vi "SetupStriptest.vi"(3 "Probe Card Channels":i32=1) -> (1 "Continue?":bool)   [LabVIEW 2018]
uses:
  ProbePlan/ProbePlanParams.vi
  general_VIs/globals/QC_RunInformation.vi
  general_VIs/globals/QC_MeasurementSetup.vi
panel:
  in  "Sensor Bias":dbl=-150.0
  out "Instructions:":string="- configure Arduino edgesense; optional testing of edgesense                                        - define probing range\n- select LCR meter, bias, and IV supply; configure if necessary                                         - adjust measurement parameters\n- select operator                                                                                                          - select tests included"
  in  "Bias Supply":u16(ring) items=["Dont set here"]
  in  "Test Button":bool
  in  "Resistance Y/N":bool=TRUE
  in  "Capacitance Y/N":bool=TRUE
  in  "Pinholes Y/N":bool=TRUE
  in  "High Step":i32=1000
  in  "Base Step":i32=1000
  in  "High Ramp":dbl=100.0
  in  "Base Ramp":dbl=10.0
  in  "High V":dbl=100.0
  in  "Base V":dbl=10.0
  in  "Quit":bool
  in  "Continue":bool
  in  "Settings Button":bool
  in  "T/RH Readout":enum16{"Arduino Uno", "Nothing"}(ring)=enum."Nothing"
  in  "LCR meter:":u16(ring) items=["Dont set here"]
  in  "IV Supply:":u16(ring) items=["Dont set here"]
  in  "Operator:":u32(ring) items=["Jiri Kv", "Saevar", "Maurice", "Rick", "Dave", "Bart", "Miguel", "Christoph", "Other..."]
  out "DataBase Serial No.:":string="DatabaseSerialNo"
  out "Manufacturer:":string="Hamamatsu"
  out "Device Category:":string
  out "Manufacturer Serial No.:":string="ManufactSerialNo"
  out "Region4":string
  out "Region3":string
  out "Region2":string
  out "Region":string
  in  "From4":u16(ring)
  in  "From3":u16(ring)
  in  "From2":u16(ring)
  in  "From":u16(ring)
  in  "To4":u16(ring)
  in  "To3":u16(ring)
  in  "To2":u16(ring)
  in  "To":u16(ring)
  in  "Enable4":bool
  in  "Enable3":bool
  in  "Enable2":bool
  in  "Enable1":bool
  # "Setup Striptest"
  # "Define Probe Range"
  # "Measurement Parameters"
  # "Volts"
  # "Base Voltage Settings"
  # "High Voltage Settings"
  # "Volts"
  # "Volts"
  # "Volts/step"
  # "Volts/step"
  # "millisec"
  # "millisec"
  # "DUT & Test Description"
  # "Tests Included"
  # "Hardware"
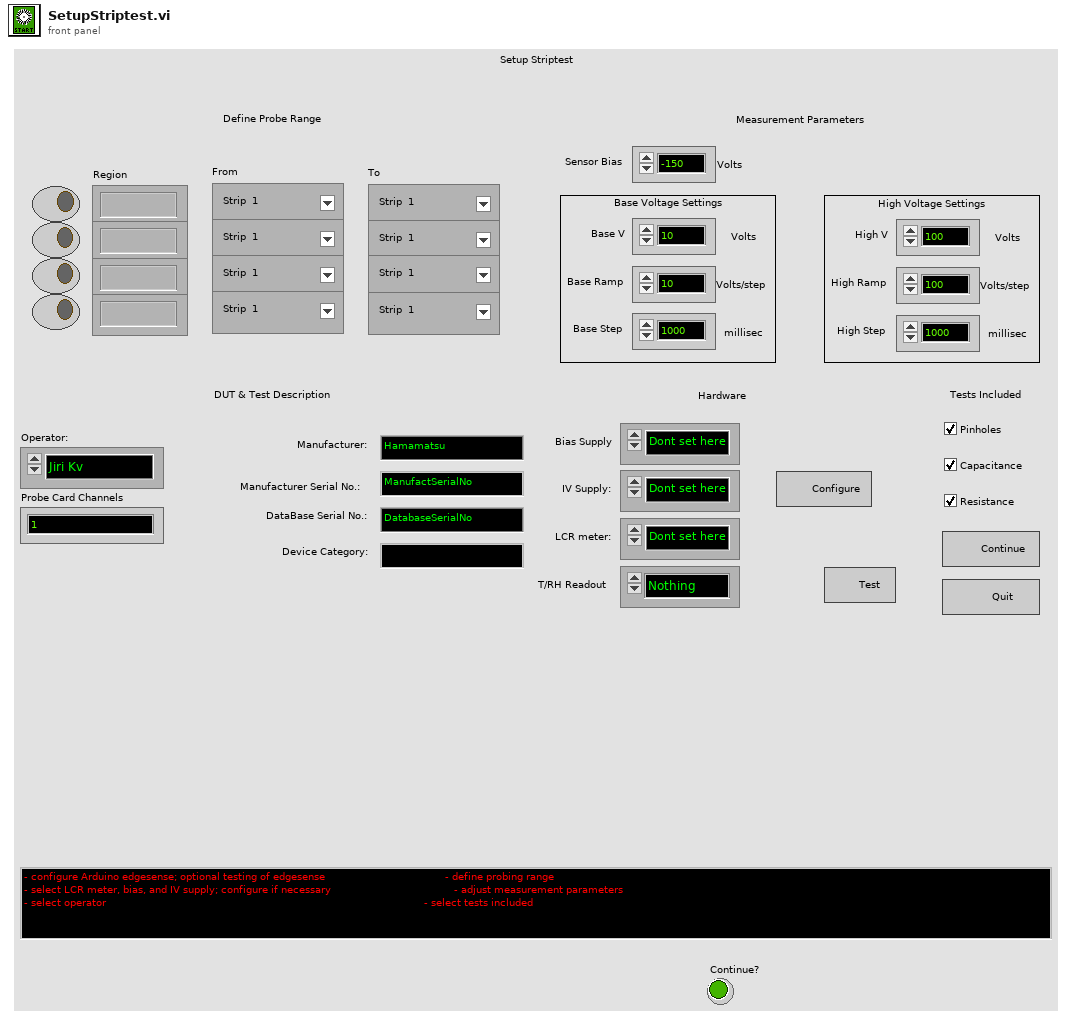
[diagram p1: front panel]
types:
  T1 = cluster{"Strip Number OUT":i32, "X0":i32, "Y0":i32, "X1":i32, "Y1":i32, "Xref":dbl, "Yref":dbl, "ProbePlan type":u32, "Inner pads offset":ext, "Outer pads offset":ext, "l_inner":ext, "l_outer":ext, "strip numbering":u16, "Device Orientation":ext, "Stagger offset":i32, "Yoffset":dbl, "Strip pitch":dbl, "Fiducail separation":dbl, "Radius":ext, "Relative strip angles":dbl, "Probeplan description":string, "ProbePlan array":cluster{"Region":string, "ProbePoints":cluster{"X":dbl, "Y":dbl, "Label":string, "CardViable?":bool}[]}[], "Test ProbePoints":cluster{"Regions Enabled":bool[], "From index":u32[], "To index":u32[]}}
  T2 = cluster{"Region":string, "ProbePoints":cluster{"X":dbl, "Y":dbl, "Label":string, "CardViable?":bool}[]}[]
  T3 = cluster{"Sensor Serial No.:":string, "Wafer Serial No.:":string, "Batch:":string, "Manufacturer:":string, "Device Category:":string, "Database Serial No.:":string, "Initiated:":string, "Test":string, "Instruments used:":string, "Probeplan used:":string, "End of Run comment:":string, "User:":string}
  T4 = cluster{"Bias Supply":refnum<class "SupplyControl.lvclass">, "SMU":refnum<class "SupplyControl.lvclass">, "LCR":refnum<class "LCRControl.lvclass">, "Probe Card Channels":i32, "Bias Voltage [V]":dbl, "First strip":i32, "Last strip":i32, "Base Voltage [V]":dbl, "Base Ramp Step [V]":dbl, "Base Ramp Interval [ms]":u32, "High Voltage [V]":dbl, "High Ramp Step [V]":dbl, "High Ramp Interval [ms]":u32, "Single Needle":bool, "Temperature Readout":enum16{"Read Arduino", "Enter manually"}, "Arduino":refnum<class "ArduinoControl.lvclass">, "Fraction of good strips [%]":dbl, "ProbeStation":refnum<class "ProbeStationControl.lvclass">, "AC frequency [Hz]":i32, "Switching":refnum<class "Switching.lvclass">, "Matrix used?":bool, "Matrix X Channels":cluster{"Bias Supply / SMU LO":i32, "Bias Supply / SMU HI":i32, "CV Box LO":i32, "CV Box HI":i32, "CV Box LO IN":i32, "CV Box HI IN":i32, "Volt meter LO":i32, "Volt meter HI":i32, "Mux1 C1":i32, "Mux1 C2":i32, "Mux2 C1":i32, "Mux2 C2":i32}, "Pinholes Y/N":bool, "Capacitance Y/N":bool, "Resistance Y/N":bool}
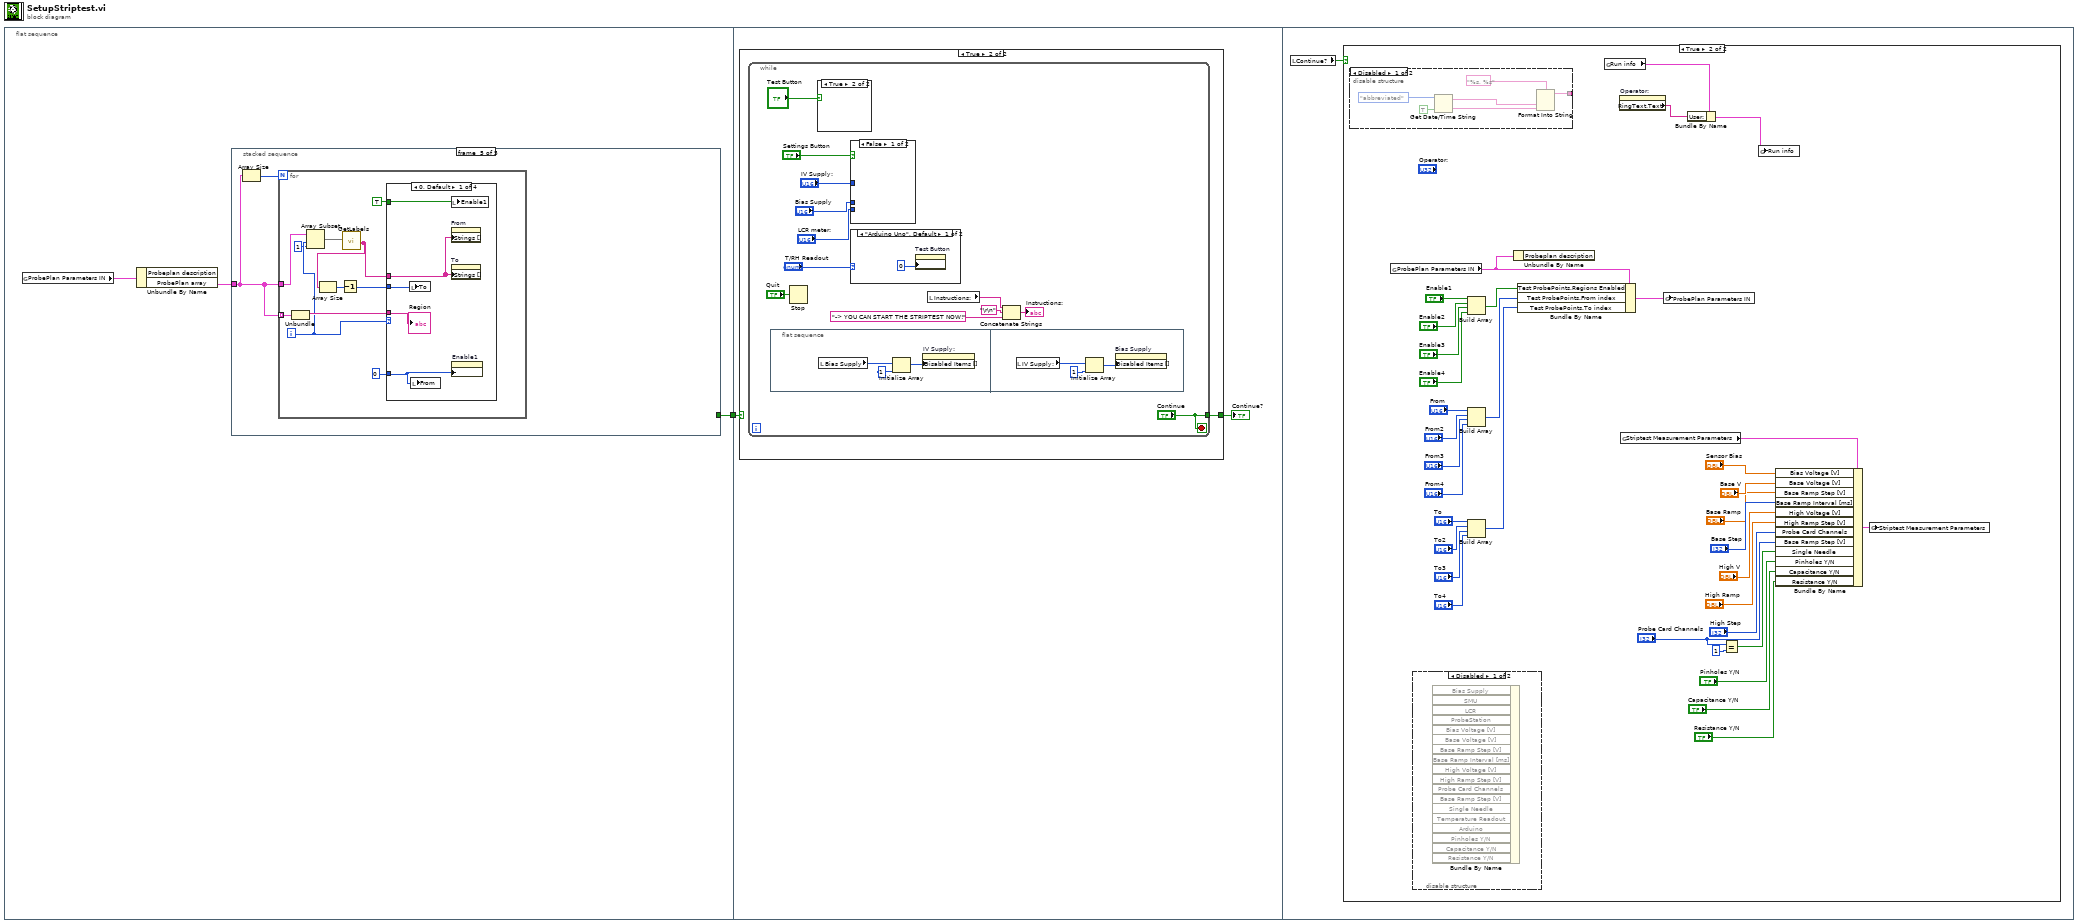
[diagram p0: block diagram]
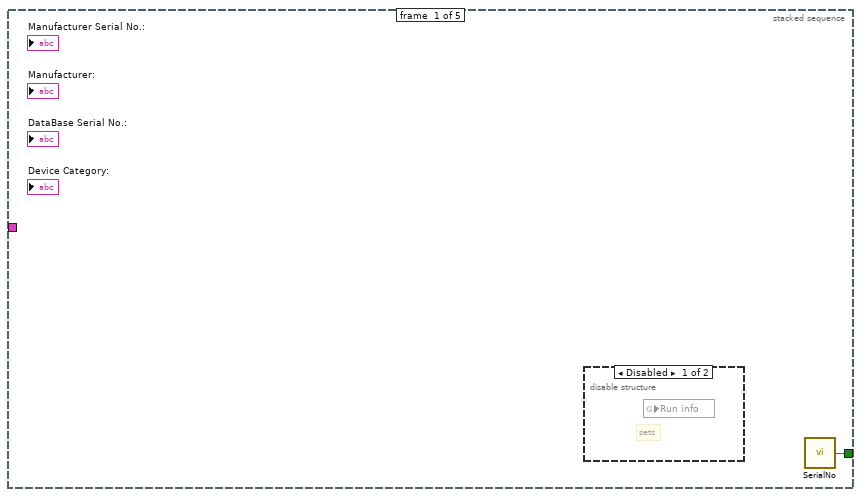
[diagram p2: hidden frame]
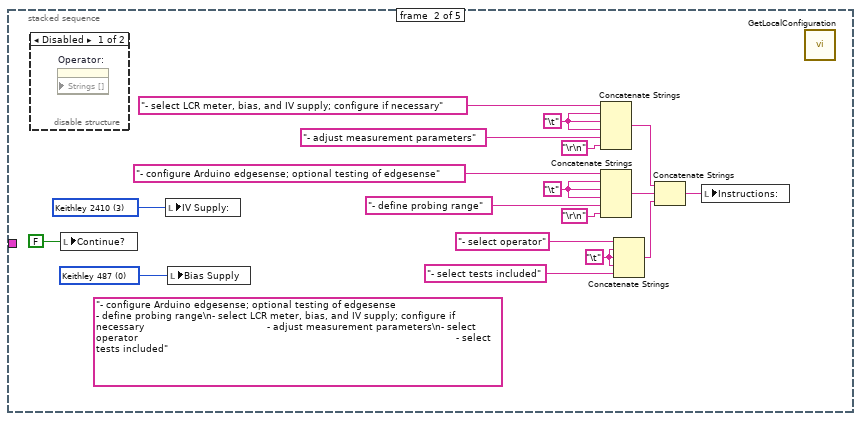
[diagram p4: hidden frame]
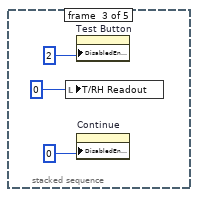
[diagram p6: hidden frame]
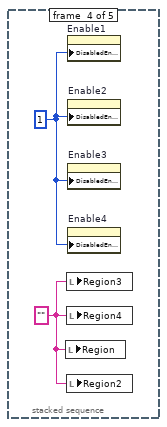
[diagram p7: hidden frame]
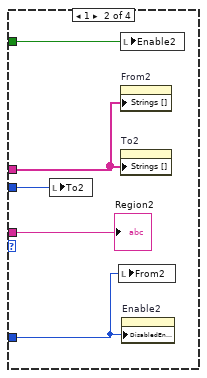
[diagram p8: hidden frame]
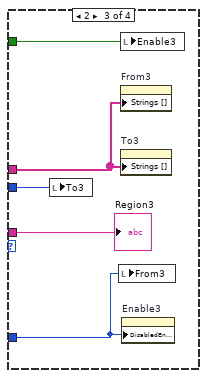
[diagram p9: hidden frame]
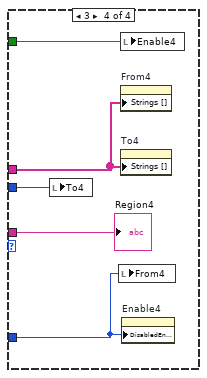
[diagram p10: hidden frame]
diagram:
  n1 = flat-sequence {
    tunnel: [w2] -> w1
    tunnel: w1 -> [w62]
    frame #0 {
      n2 = global read "ProbePlanParams.vi" "ProbePlan Parameters IN"() -> (w4:T1)
      n3 = Unbundle By Name(w4) -> ("ProbePlan array"=w3:T2)  [unwired: 1 out]
      n4 = stacked-sequence {
        tunnel: w3 -> [_ _ _ _ w29]
        tunnel: [w5 _ _ _ _] -> w2
        frame #0 {
          n5 = disable-structure shown="Disabled" {
            frame Disabled {
              # "sets"
              n6 = global read "QC_RunInformation.vi" "Run info"() -> ()  [unwired: 1 in]
            }
            frame Enabled {
            }
          }
          n7 = call "SerialNo.vi"() -> ("Continue?"=w5:bool)  [unwired: 5 in]
        }
        frame #1 {
          w14 = "\t"
          w16 = "\t"
          w20 = "\t"
          (unwired) "- configure Arduino edgesense; optional testing of edgesense                                        - define probing range\n- select LCR meter, bias, and IV supply; configure if necessary                                         - adjust measurement parameters\n- select operator                                                                                                          - select tests included" ("Instructions:")
          w21 = u16 0 items=["Keithley 487", "Keithley 6517", "Keithley 236/237", "Keithley 2410"] ("Supply:")
          w22 = u16 3 items=["Keithley 487", "Keithley 6517", "Keithley 236/237", "Keithley 2410"] ("Supply:")
          n8 = disable-structure shown="Disabled" {
            frame Disabled {
              n9 = property on="Operator:" class="Ring (strict)" props=["Strings []"]() -> ()  [unwired: 3 in, 2 out]
            }
            frame Enabled {
            }
          }
          n10 = local write "Continue?"(FALSE ("Continue?")) -> ()
          n11 = local write "IV Supply:"(w22) -> ()
          n12 = local write "Bias Supply"(w21) -> ()
          n13 = Concatenate Strings("- select LCR meter, bias, and IV supply; configure if necessary", w16, w16, w16, "- adjust measurement parameters", "\r\n") -> (w9:string)
          n14 = Concatenate Strings("- configure Arduino edgesense; optional testing of edgesense", w20, w20, w20, "- define probing range", "\r\n") -> (w10:string)
          n15 = Concatenate Strings("- select operator", w14, w14, w14, "- select tests included") -> (w11:string)
          n16 = Concatenate Strings(w9, w10, w11) -> (w8:string)
          n17 = local write "Instructions:"(w8) -> ()
          n18 = call "GetLocalConfiguration.vi"() -> ()  [unwired: 3 in, 1 out]
        }
        frame #2 {
          n19 = local write "T/RH Readout"(0) -> ()
          n20 = property on="Test Button" class="Bool"("DisabledEnum"=2) -> ()  [unwired: 2 in, 2 out]
          n21 = property on="Continue" class="Bool"("DisabledEnum"=u8 0 ("Disabled")) -> ()  [unwired: 2 in, 2 out]
        }
        frame #3 {
          w28 = "" ("Region")
          w27 = u8 1 ("Disabled")
          n22 = local write "Region"(w28) -> ()
          n23 = local write "Region3"(w28) -> ()
          n24 = local write "Region4"(w28) -> ()
          n25 = local write "Region2"(w28) -> ()
          n26 = property on="Enable1" class="Bool (strict)"("DisabledEnum"=w27) -> ()  [unwired: 2 in, 2 out]
          n27 = property on="Enable2" class="Bool (strict)"("DisabledEnum"=w27) -> ()  [unwired: 2 in, 2 out]
          n28 = property on="Enable3" class="Bool (strict)"("DisabledEnum"=w27) -> ()  [unwired: 2 in, 2 out]
          n29 = property on="Enable4" class="Bool (strict)"("DisabledEnum"=w27) -> ()  [unwired: 2 in, 2 out]
        }
        frame #4 {
          n30 = Array Size(array=w29) -> (size(s)=w30:i32)
          n31 = for {
            N: w30 -> [_]
            tunnel: w29 -> [w34]
            tunnel: w29 -> [w39] mode=indexing
            i -> [w33]
            n32 = Unbundle(w39) -> ("Region"=w38:string)  [unwired: 1 out]
            n33 = Array Subset(array=w34, index=w33, length=1) -> (w31:T2)
            n34 = call "GetLabels.vi"("Array"=w31) -> ("Strip Labels"=w35:string[])  [unwired: 3 out]
            n35 = Array Size(array=w35) -> (size(s)=w37:i32)
            n36 = Decrement(x=w37) -> (x-1=w36:i32)
            n37 = case shown="0, Default" w33 {
              tunnel: TRUE -> [w46 w50 w56 w61]
              tunnel: 0 -> [w42 w47 w52 w57]
              tunnel: w38 -> [w44 w49 w54 w59]
              tunnel: w35 -> [w43 w48 w53 w58]
              tunnel: w36 -> [w45 w51 w55 w60]
              frame 0, Default {
                n38 = local write "To"(w45) -> ()
                n39 = local write "From"(w42) -> ()
                n40 = local write "Enable1"(w46) -> ()
                n41 = property on="From" class="Ring (strict)"("Strings []"=w43) -> ()  [unwired: 2 in, 2 out]
                n42 = property on="To" class="Ring (strict)"("Strings []"=w43) -> ()  [unwired: 2 in, 2 out]
                n43 = property on="Enable1" class="Bool (strict)"("DisabledEnum"=w42) -> ()  [unwired: 2 in, 2 out]
                "Region" <- w44
              }
              frame 1 {
                n44 = local write "To2"(w51) -> ()
                n45 = local write "From2"(w47) -> ()
                n46 = local write "Enable2"(w50) -> ()
                n47 = property on="From2" class="Ring (strict)"("Strings []"=w48) -> ()  [unwired: 2 in, 2 out]
                n48 = property on="To2" class="Ring (strict)"("Strings []"=w48) -> ()  [unwired: 2 in, 2 out]
                n49 = property on="Enable2" class="Bool (strict)"("DisabledEnum"=w47) -> ()  [unwired: 2 in, 2 out]
                "Region2" <- w49
              }
              frame 2 {
                n50 = local write "To3"(w55) -> ()
                n51 = local write "From3"(w52) -> ()
                n52 = local write "Enable3"(w56) -> ()
                n53 = property on="From3" class="Ring (strict)"("Strings []"=w53) -> ()  [unwired: 2 in, 2 out]
                n54 = property on="To3" class="Ring (strict)"("Strings []"=w53) -> ()  [unwired: 2 in, 2 out]
                n55 = property on="Enable3" class="Bool (strict)"("DisabledEnum"=w52) -> ()  [unwired: 2 in, 2 out]
                "Region3" <- w54
              }
              frame 3 {
                n56 = local write "To4"(w60) -> ()
                n57 = local write "From4"(w57) -> ()
                n58 = local write "Enable4"(w61) -> ()
                n59 = property on="From4" class="Ring (strict)"("Strings []"=w58) -> ()  [unwired: 2 in, 2 out]
                n60 = property on="To4" class="Ring (strict)"("Strings []"=w58) -> ()  [unwired: 2 in, 2 out]
                n61 = property on="Enable4" class="Bool (strict)"("DisabledEnum"=w57) -> ()  [unwired: 2 in, 2 out]
                "Region4" <- w59
              }
            }
          }
        }
      }
    }
    frame #1 {
      n62 = case shown="True" w62 {
        selector: w62 -> [w64 _]
        tunnel: [w64 w65] -> w63
        frame False {
        }
        frame True {
          n63 = while {
            tunnel: ["Continue"] -> w65
            stop <- "Continue" stop-if-true
            n64 = flat-sequence {
              frame #0 {
                n65 = local read "Bias Supply"() -> (w79:u16)
                n66 = Initialize Array(w79, 1) -> (w80:u16[])
                n67 = property on="IV Supply:" class="Ring (strict)"("Disabled Items []"=w80) -> ()  [unwired: 2 in, 2 out]
              }
              frame #1 {
                n68 = local read "IV Supply:"() -> (w84:u16)
                n69 = Initialize Array(w84, 1) -> (w82:u16[])
                n70 = property on="Bias Supply" class="Ring (strict)"("Disabled Items []"=w82) -> ()  [unwired: 2 in, 2 out]
              }
            }
            n71 = Stop(stop? (T)="Quit") -> ()
            n72 = case shown="True" "Test Button" {
              frame False {
              }
              frame True {
              }
            }
            n73 = case shown="False" "Settings Button" {
              tunnel: "IV Supply:" -> [_ _]
              tunnel: "LCR meter:" -> [_ _]
              tunnel: "Bias Supply" -> [_ _]
              frame False {
              }
              frame True {
              }
            }
            n74 = case shown="\"Arduino Uno\", Default" "T/RH Readout" {
              frame "Arduino Uno", Default {
                n75 = property on="Test Button" class="Bool"("DisabledEnum"=0) -> ()  [unwired: 2 in, 2 out]
              }
              frame "Nothing" {
              }
            }
            n76 = local read "Instructions:"() -> (w68:string)
            n77 = Concatenate Strings(w68, "\r\n", "-> YOU CAN START THE STRIPTEST NOW!") -> (→"Instructions:":string)
          }
        }
      }
      "Continue?" <- w63
    }
    frame #2 {
      n78 = local read "Continue?"() -> (w85:bool)
      n79 = case shown="True" w85 {
        frame False {
        }
        frame True {
          n80 = disable-structure shown="Disabled" {
            disable-tunnel: [w121 _] -> _
            frame Disabled {
              n81 = Get Date/Time String(date format (0)=enum16{"short", "long", "abbreviated"}."abbreviated", want seconds? (F)=TRUE) -> (date string=w123:string, time string=w122:string)  [unwired: 1 in]
              n82 = Format Into String(format string="%s, %s", w123, w122) -> (resulting string=w121:string)  [unwired: 2 in, 1 out]
            }
            frame Enabled {
            }
          }
          n83 = global read "ProbePlanParams.vi" "ProbePlan Parameters IN"() -> (w98:T1)
          n84 = disable-structure shown="Disabled" {
            frame Disabled {
              n85 = Bundle By Name() -> ()  [unwired: 19 in, 1 out]
            }
            frame Enabled {
            }
          }
          n86 = Build Array("Enable1", "Enable2", "Enable3", "Enable4") -> (w106:bool[])
          n87 = Build Array("From", "From2", "From3", "From4") -> (w107:u16[])
          n88 = Build Array("To", "To2", "To3", "To4") -> (w108:u16[])
          n89 = Unbundle By Name(w98) -> ()  [unwired: 1 out]
          n90 = Bundle By Name(cluster=w98, "Test ProbePoints.Regions Enabled"=w106, "Test ProbePoints.From index"=w107, "Test ProbePoints.To index"=w108) -> (w105:T1)
          n91 = global read "QC_RunInformation.vi" "Run info"() -> (w93:T3)
          n92 = property on="Operator:" class="Ring (strict)"() -> ("RingText.Text"=w86:string)  [unwired: 2 in, 2 out]
          n93 = global read "QC_MeasurementSetup.vi" "Striptest Measurement Parameters"() -> (w87:T4)
          n94 = global write "ProbePlanParams.vi" "ProbePlan Parameters IN"(w105) -> ()
          n95 = Bundle By Name(cluster=w93, "User:"=w86) -> (w94:T3)
          n96 = Equal?(x="Probe Card Channels", y=1) -> (x = y?=w95:bool)
          n97 = global write "QC_RunInformation.vi" "Run info"(w94) -> ()
          n98 = Bundle By Name(cluster=w87, "Bias Voltage [V]"="Sensor Bias", "Base Voltage [V]"="Base V", "Base Ramp Step [V]"="Base Ramp", "Base Ramp Interval [ms]"="Base Step", "High Voltage [V]"="High V", "High Ramp Step [V]"="High Ramp", "Probe Card Channels"="High Step", "Base Ramp Step [V]"="Probe Card Channels", "Single Needle"=w95, "Pinholes Y/N"="Pinholes Y/N", "Capacitance Y/N"="Capacitance Y/N", "Resistance Y/N"="Resistance Y/N") -> (w92:T4)
          n99 = global write "QC_MeasurementSetup.vi" "Striptest Measurement Parameters"(w92) -> ()
        }
      }
    }
  }
